vi "covertnumbervi.vi"(7 "error in":errorcluster, 9 "Array":string[](array[string])) -> (0 "error out":errorcluster, 1 "Symbol":string, 2 "Array Out":dbl[](array[numeric]), 3 "max value":dbl, 4 "min value":dbl)   [LabVIEW 2022 SP3]
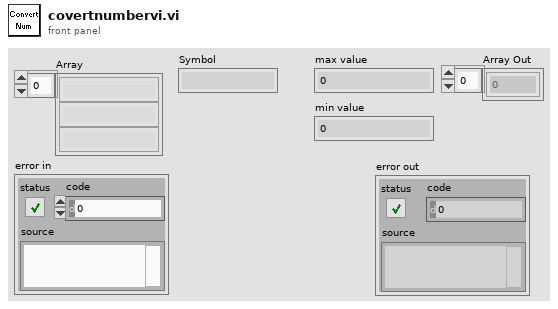
[diagram p1: front panel]
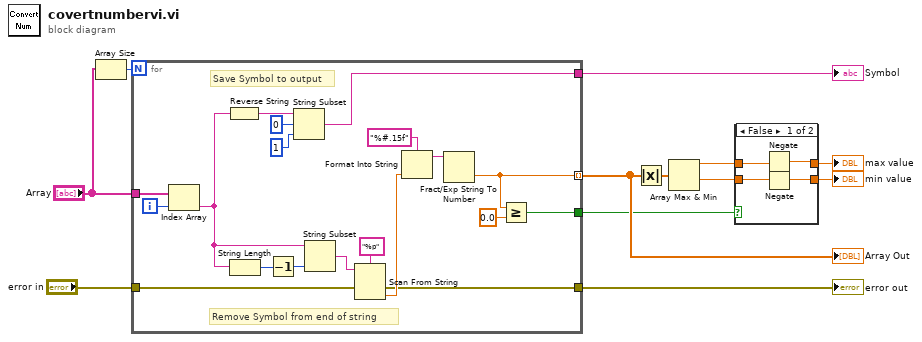
[diagram p0: block diagram]
diagram:
  n1 = Array Size(array="Array") -> (size(s)=w12:i32)
  n2 = for {
    N: w12 -> [_]
    tunnel: "Array" -> [w24]
    tunnel: [w22] -> w10
    tunnel: [w14] -> w7 mode=indexing
    tunnel: "error in" -> [w17]
    tunnel: [w16] -> w8
    tunnel: [w13] -> w6
    i -> [w25]
    # "Save Symbol to output"
    # "Remove Symbol from end of string"
    n3 = Index Array(array=w24, index=w25) -> (element=w23:string)
    n4 = Reverse String(1:w23) -> (0:w26:string)
    n5 = String Length(string=w23) -> (length=w30:i32)
    n6 = Decrement(x=w30) -> (x-1=w29:i32)
    n7 = String Subset(string=w26, offset (0)=0 ("index"), length (rest)=1 ("length (rest)")) -> (substring=w22:string)
    n8 = String Subset(string=w23, length (rest)=w29) -> (substring=w21:string)  [unwired: 1 in]
    n9 = Scan From String(format string="%p", input string=w21, error in=w17) -> (error out=w16:errorcluster, output 1=w20:dbl)  [unwired: 2 in, 2 out]
    n10 = Format Into String(format string="%#.15f", w20) -> (resulting string=w18:string)  [unwired: 2 in, 1 out]
    n11 = Fract/Exp String To Number(string=w18) -> (number=w14:dbl)  [unwired: 3 in, 1 out]
    n12 = Greater Or Equal?(x=w14, y=0.0) -> (x >= y?=w13:bool)
  }
  "Symbol" <- w10
  "error out" <- w8
  "Array Out" <- w7
  n13 = Absolute Value(x=w7) -> (abs(x)=w1:dbl[])
  n14 = Array Max & Min(array=w1) -> (max value=w5:dbl, min value=w4:dbl)  [unwired: 2 out]
  n15 = case shown="False" w6 {
    tunnel: [w33 w37] -> w3
    tunnel: w5 -> [w35 w37]
    tunnel: [w32 w36] -> w2
    tunnel: w4 -> [w34 w36]
    frame False {
      n16 = Negate(x=w35) -> (-x=w33:dbl)
      n17 = Negate(x=w34) -> (-x=w32:dbl)
    }
    frame True {
    }
  }
  "min value" <- w2
  "max value" <- w3
